vi "U3 ms Multiple Pulse Output.vi"() -> ()   [LabVIEW 2021]
panel:
  in  "Number of Pulses":dbl=1.0 min=1.0 format="%.2f"
  in  "Pulse Width (ms)":dbl=10.0 min=0.004 format="%.3f"
  in  "FirstFound":bool=TRUE
  in  "Address":string="1"
  out "Error Message":string
  # "Demonstrates using a PWM output (FIO4) and a stop timer (FIO5) to create multiple pulses with\na pulse width from 0.004-262 ms which is variable in 4 us increments.  \n\nA jumper must be installed from FIO4 to FIO5 for the stop timer to work.\n\nThe pulses are negative (signal is normally-high).  If positive pulses are needed, an inverter IC\nshould be put on the signal.\n\nFrequency of the pulses is 3.8 Hz.  PWM output (and frequency output) does not necessarily\nstart instantly, but rather waits for the internal clock to roll.  With a frequency of 3.8 Hz, the\nperiod is 262 ms, so after the command is received by the U3, it could be anywhere\nfrom 0 to 262 ms before the start of the first low time of the first PWM cycle."
  # "This VI passes a timer\nbase clock constant that\nis valid for hardware V1.21.\nFor hardware V1.20 change\nLJ_tc48MHZ to LJ_tc24MHZ."
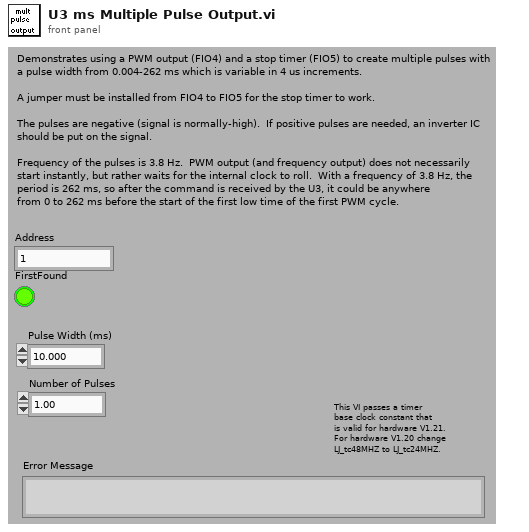
[diagram p1: front panel]
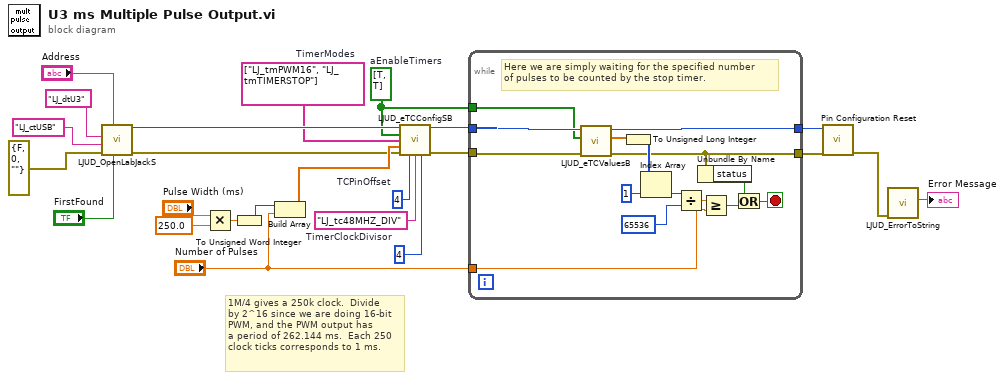
[diagram p0: block diagram]
diagram:
  w3 = 4  # TimerClockDivisor
  w5 = 4  # TCPinOffset
  w2 = bool[] [TRUE, TRUE]  # aEnableTimers
  w6 = string[] ["LJ_tmPWM16", "LJ_tmTIMERSTOP"]  # TimerModes
  # "1M/4 gives a 250k clock.  Divide\nby 2^16 since we are doing 16-bit\nPWM, and the PWM output has\na period of 262.144 ms.  Each 250\nclock ticks corresponds to 1 ms."
  n1 = call "LJUD_OpenLabJackS.vi"("FirstFound"="FirstFound", "Address"="Address", "error in"=errorcluster {"status"=FALSE, "code"=0, "source"=""}, "ConnectionType"="LJ_ctUSB", "DeviceType"="LJ_dtU3") -> ("error out"=w8:errorcluster, "Handle"=w7:i32)  [unwired: 4 in, 1 out]
  n2 = Multiply(x="Pulse Width (ms)", y=250.0) -> (x*y=w15:dbl)
  n3 = To Unsigned Word Integer(number=w15) -> (unsigned 16bit integer=w12:u16)
  n4 = Build Array(w12, "Number of Pulses") -> (w14:dbl[])
  n5 = call "LJUD_eTCConfigSB.vi"("Handle In"=w7, "aEnableTimers"=w2, "aTimerModes"=w6, "aTimerValues"=w14, "error in"=w8, "TCPinOffset"=w5, "TimerClockBase"="LJ_tc48MHZ_DIV" ("Timer Clock Base"), "TimerClockDivisor"=w3) -> ("Handle Out"=w10:i32, "error out"=w11:errorcluster)  [unwired: 6 in]
  n6 = while {
    tunnel: w2 -> [w29]
    tunnel: "Number of Pulses" -> [w30]
    tunnel: w11 -> [w37]
    tunnel: w10 -> [w38]
    tunnel: [w39] -> w21
    tunnel: [w26] -> w9
    stop <- w25 stop-if-true
    # "Here we are simply waiting for the specified number\nof pulses to be counted by the stop timer."
    n7 = call "LJUD_eTCValuesB.vi"("error in"=w37, "aReadTimers"=w29, "Handle In"=w38) -> ("error out"=w26:errorcluster, "aTimerValues Read"=w33:dbl[], "Handle Out"=w39:i32)  [unwired: 5 in, 1 out]
    n8 = To Unsigned Long Integer(number=w33) -> (unsigned 32bit integer=w32:u32[])
    n9 = Index Array(array=w32, index=1 ("Index")) -> (element=w34:u32)
    n10 = Divide(x=w34, y=u32 65536) -> (x/y=w35:dbl)
    n11 = Unbundle By Name(w26) -> ("status"=w27:bool)
    n12 = Greater Or Equal?(x=w35, y=w30) -> (x >= y?=w28:bool)
    n13 = Or(x=w27, y=w28) -> (x .or. y?=w25:bool)
  }
  n14 = call "Pin Configuration Reset.vi"("error in"=w9, "Handle In"=w21) -> ("error out"=w20:errorcluster)  [unwired: 8 in, 1 out]
  n15 = call "LJUD_ErrorToString.vi"("error in"=w20) -> ("String"=→"Error Message":string)  [unwired: 10 in]
